vi "Main.vi"() -> ()   [LabVIEW 2020]
uses:
  Clases/Abstracta/Camara/Camara.lvclass
panel:
  out "Image":T1(plugin-control)
  in  "Stop":bool
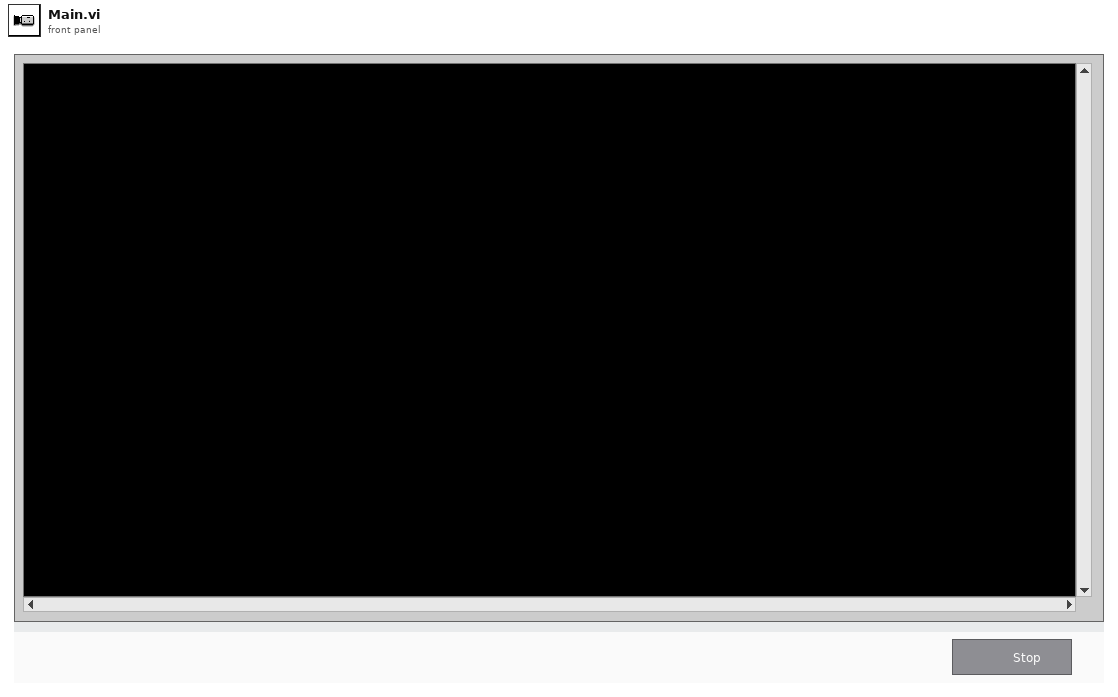
[diagram p1: front panel]
types:
  T1 = typedef "IMAQ Image.ctl" = refnum<image>
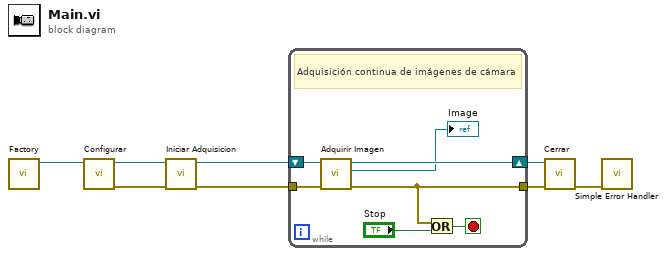
[diagram p0: block diagram]
diagram:
  n1 = call "Factory.vi"() -> ("specific class reference"=w2:refnum<class "Camara.lvclass">)  [unwired: 11 in]
  n2 = call-dynamic "Configurar.vi"("Camara in"=w2) -> ("error out"=w7:errorcluster, "Camara out"=w8:refnum<class "Camara.lvclass">)  [unwired: 9 in]
  n3 = call-dynamic "Iniciar Adquisicion.vi"("error in (no error)"=w7, "Camara in"=w8) -> ("error out"=w5:errorcluster, "Camara out"=w6:refnum<class "Camara.lvclass">)  [unwired: 8 in]
  n4 = while {
    shift-right: [w13] -> w4
    shift-left: w6 -> [w15]
    tunnel: w5 -> [w14]
    tunnel: [w10] -> w3
    stop <- w11 stop-if-true
    # "Adquisición continua de imágenes de cámara"
    n5 = call-dynamic "Adquirir Imagen.vi"("error in (no error)"=w14, "Camara in"=w15) -> ("error out"=w10:errorcluster, "Imagen"=→"Image":T1, "Camara out"=w13:refnum<class "Camara.lvclass">)  [unwired: 7 in]
    n6 = Or(x=w10, y="Stop") -> (x .or. y?=w11:bool)
  }
  n7 = call-dynamic "Cerrar.vi"("error in (no error)"=w3, "Camara in"=w4) -> ("error out"=w1:errorcluster)  [unwired: 8 in, 1 out]
  n8 = call <vilib>:"Simple Error Handler.vi"("error in (no error)"=w1) -> ()  [unwired: 4 in, 5 out]
